vi "dfd_DFXPSimu AccSub (scaler).vi"(5 "quantize output?(T)":bool=TRUE, 7 "op params":T1={"source"=0, "is floating?"=FALSE, "o-mode"=enum."Wrap", "q-mode"=enum."Truncation", "wl"=1, "high limit"=0, "low limit"=0, "iwl"=0, "sign?"=TRUE} {"source" items=["Coef a/k"=0, "Coef b/v"=7, "Input"=1, "Output"=2, "Multiplicand"=3, "Product"=4, "Sum"=5, "Delay"=6, "Gain"=8]}, 8 "filtering statistics in":T5(array[cluster]) {"statistics information"."min value" format="%.2f"; "statistics information"."max value" format="%.2f"; "Quantizer Source" items=["Coefficients a/k"=0, "Coefficients b/v"=7, "Input"=1, "Output"=2, "Multiplicand"=3, "Product"=4, "Sum"=5, "Delay"=6]}, 10 "addend":T6={"value"=0, "wl"=0, "iwl"=0, "Signed"=TRUE} {"value" format="%.0x"}, 11 "acc in":T6={"value"=0, "wl"=0, "iwl"=0, "Signed"=TRUE} {"value" format="%.0x"}) -> (0 "filtering statistics out":T5(array[cluster]) {"statistics information"."min value" format="%.2f"; "statistics information"."max value" format="%.2f"; "Quantizer Source" items=["Coefficients a/k"=0, "Coefficients b/v"=7, "Input"=1, "Output"=2, "Multiplicand"=3, "Product"=4, "Sum"=5, "Delay"=6]}, 3 "acc out":T6={"value"=0, "wl"=0, "iwl"=0, "Signed"=TRUE} {"value" format="%.0x"})   [LabVIEW 2017, in "NI_DigFilter_FXP.lvlib"]
uses:
  <vilib>/addons/Digital Filter Design/NI_DigFilter_FXP.lvlib
  <vilib>/addons/Digital Filter Design/_Objects.llb/dfd_DFXP Data Type (scaler).ctl
  <vilib>/addons/Digital Filter Design/_Objects.llb/DFD Quantization Sources.ctl
  <vilib>/addons/Digital Filter Design/_Objects.llb/DFD FXP Statistics Data.ctl
  <vilib>/addons/Digital Filter Design/_Objects.llb/dfd_DFXP Operation Parameter.ctl
  <vilib>/addons/Digital Filter Design/_Objects.llb/dfd_Internal Quantization Srcs.ctl
  <vilib>/addons/Digital Filter Design/NI_DigFilterLicensed.lvlib
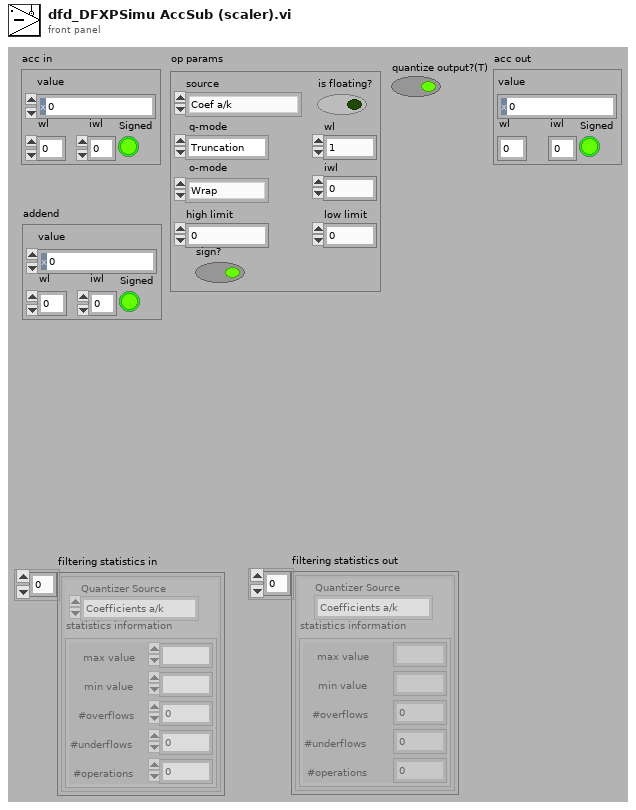
[diagram p1: front panel]
types:
  T1 = typedef "dfd_DFXP Operation Parameter.ctl" = cluster{"source":T2, "is floating?":bool, "o-mode":enum16{"Saturation", "Wrap"}, "q-mode":enum16{"Nearest", "Truncation"}, "wl":i16, "high limit":i64, "low limit":i64, "iwl":i16, "sign?":bool}
  T2 = typedef "NI_DigFilterLicensed.lvlib/dfd_Internal Quantization Srcs.ctl" = u16
  T3 = typedef "NI_DigFilterLicensed.lvlib/DFD Quantization Sources.ctl" = u16
  T4 = typedef "NI_DigFilterLicensed.lvlib/DFD FXP Statistics Data.ctl" = cluster{"max value":ext, "min value":ext, "#overflows":i32, "#underflows":i32, "#operations":i32}
  T5 = cluster{"Quantizer Source":T3, "statistics information":T4}[]
  T6 = typedef "dfd_DFXP Data Type (scaler).ctl" = cluster{"value":i64, "wl":i16, "iwl":i16, "Signed":bool}
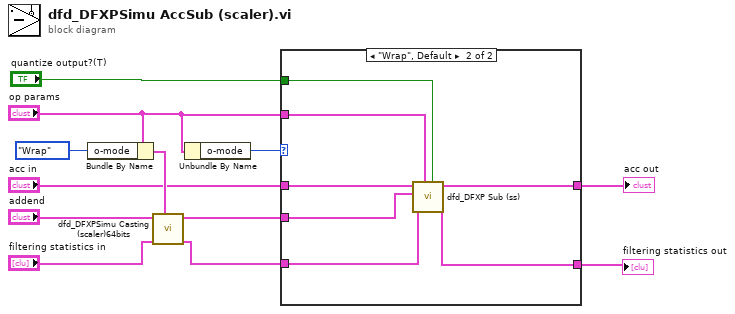
[diagram p0: block diagram]
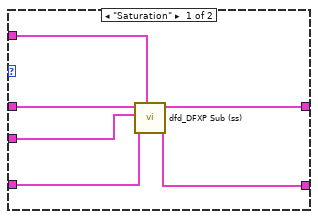
[diagram p2: hidden frame]
diagram:
  n1 = Bundle By Name(cluster="op params", "o-mode"=enum16{"Saturation", "Wrap"}."Wrap" ("o_mode")) -> (w10:T1)
  n2 = call <vilib>:"dfd_DFXPSimu Casting (scaler)64bits.vi"("op params"=w10, "filtering statistics in"="filtering statistics in", "Value in"="addend") -> ("filtering statistics out"=w4:T5, "Value out"=w6:T6)  [unwired: 1 in, 6 out]
  n3 = Unbundle By Name("op params") -> ("o-mode"=w8:enum16{"Saturation", "Wrap"})
  n4 = case shown="\"Wrap\", Default" w8 {
    tunnel: [w18 w23] -> w2
    tunnel: [w15 w21] -> w3
    tunnel: w4 -> [w17 w22]
    tunnel: "quantize output?(T)" -> [_ w25]
    tunnel: "op params" -> [w16 w24]
    tunnel: w6 -> [w13 w19]
    tunnel: "acc in" -> [w14 w20]
    frame "Saturation" {
      n5 = call <vilib>:"dfd_DFXP Sub (ss).vi"("op params"=w16, "filtering statistics in"=w17, "Value in 2"=w13, "Value in"=w14) -> ("filtering statistics out"=w15:T5, "Value out"=w18:T6)  [unwired: 1 in, 5 out]
    }
    frame "Wrap", Default {
      n6 = call <vilib>:"dfd_DFXP Sub (ss).vi"("quantize output?(T)"=w25, "op params"=w24, "filtering statistics in"=w22, "Value in 2"=w19, "Value in"=w20) -> ("filtering statistics out"=w21:T5, "Value out"=w23:T6)  [unwired: 5 out]
    }
  }
  "acc out" <- w2
  "filtering statistics out" <- w3
